vi "preprocessLaserReading.vi"(4 "Right Now":timestamp, 6 "Last 10 Rising Edges":timestamp[](array[timestamp]), 7 "Laser On?":bool, 9 "Reset":bool, 10 "Rising Edge?":bool, 11 "Count":u32) -> (3 "Laser Reading":T1)   [LabVIEW 2017]
uses:
  TypeDefs/laserReading.ctl
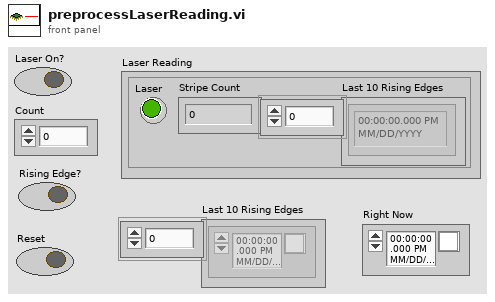
[diagram p1: front panel]
types:
  T1 = typedef "laserReading.ctl" = cluster{"Laser":bool, "Stripe Count":u32, "Last 10 Rising Edges":timestamp[]}
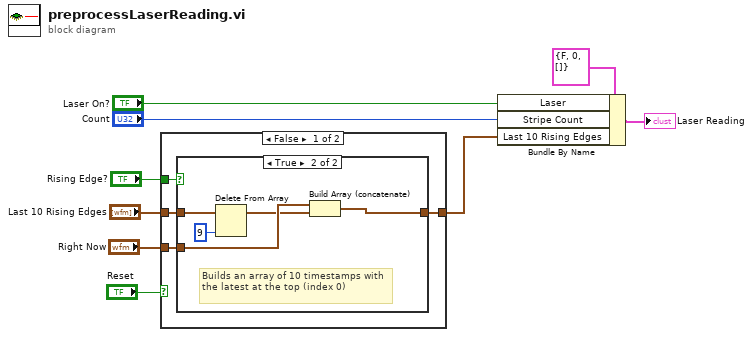
[diagram p0: block diagram]
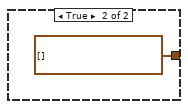
[diagram p3: hidden frame]
diagram:
  n1 = case shown="False" "Reset" {
    tunnel: "Rising Edge?" -> [w13 _]
    tunnel: [w12 timestamp[] [] ("Last 10 Rising Edges")] -> w4
    tunnel: "Last 10 Rising Edges" -> [w11 _]
    tunnel: "Right Now" -> [w10 _]
    frame False {
      n2 = case shown="True" w13 {
        tunnel: [w14 w16] -> w12
        tunnel: w11 -> [w14 w19]
        tunnel: w10 -> [_ w18]
        frame False {
        }
        frame True {
          # "Builds an array of 10 timestamps with the latest at the top (index 0)"
          n3 = Delete From Array(array=w19, index=9) -> (array with subset deleted=w17:timestamp[])  [unwired: 1 in, 1 out]
          n4 = Build Array (concatenate)(w18, w17) -> (w16:timestamp[])
        }
      }
    }
    frame True {
    }
  }
  n5 = Bundle By Name(cluster=T1 {"Laser"=FALSE, "Stripe Count"=0, "Last 10 Rising Edges"=[]} ("Laser Reading"), "Laser"="Laser On?", "Stripe Count"="Count", "Last 10 Rising Edges"=w4) -> (→"Laser Reading":T1)
